vi "TCL Get Valid Baseline.vi"(1 "RFMod (kHz)":i32, 2 "RFFreq (MHz)":dbl format="%.2f", 3 "Baseline Event #":i32) -> (0 "Baseline":dbl[](array[numeric]) format="%.2f")   [LabVIEW 2009]
doc: "This VI looks up the requested event number and then compares its rf frequency and modulation with the input values. If the event is found, and if the frequency and modulation match, the raw signal of the baseline is returned. Otherwise, an empty array is returned."
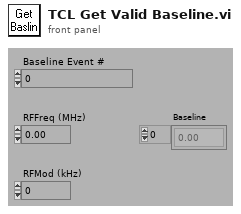
[diagram p1: front panel]
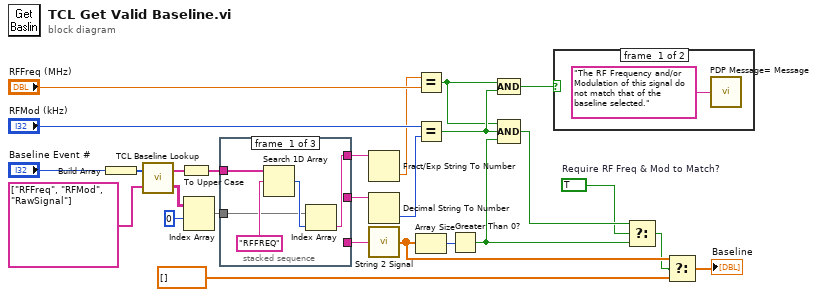
[diagram p0: block diagram]
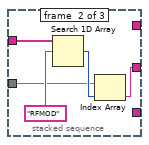
[diagram p3: hidden frame]
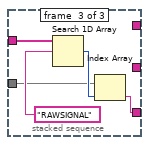
[diagram p4: hidden frame]
diagram:
  w4 = TRUE  # Require RF Freq & Mod to Match?
  n1 = Build Array("Baseline Event #") -> (w13:i32[])
  n2 = call "TCL Baseline Lookup.vi"("Fragments Desired"=string[] ["RFFreq", "RFMod", "RawSignal"], "Events Requested"=w13) -> ("Data"=w12:string[][], "Fragments Returned"=w11:string[])
  n3 = To Upper Case(1:w11) -> (0:w25:string[])
  n4 = Index Array(array=w12, index (row)=0) -> (element=w22:string[])  [unwired: 1 in]
  n5 = stacked-sequence {
    tunnel: w25 -> [w31 w36 w41]
    tunnel: w22 -> [w28 w33 w38]
    tunnel: [w27 _ _] -> w21
    tunnel: [_ w32 _] -> w23
    tunnel: [_ _ w37] -> w24
    frame #0 {
      n6 = Search 1D Array(1D array=w31, element="RFFREQ") -> (index of element=w29:i32)  [unwired: 1 in]
      n7 = Index Array(array=w28, index=w29) -> (element=w27:string)
    }
    frame #1 {
      n8 = Search 1D Array(1D array=w36, element="RFMOD") -> (index of element=w34:i32)  [unwired: 1 in]
      n9 = Index Array(array=w33, index=w34) -> (element=w32:string)
    }
    frame #2 {
      n10 = Search 1D Array(1D array=w41, element="RAWSIGNAL") -> (index of element=w39:i32)  [unwired: 1 in]
      n11 = Index Array(array=w38, index=w39) -> (element=w37:string)
    }
  }
  n12 = Fract/Exp String To Number(string=w21) -> (number=w16:dbl)  [unwired: 3 in, 1 out]
  n13 = Decimal String To Number(string=w23) -> (number=w15:i32)  [unwired: 2 in, 1 out]
  n14 = call "String 2 Signal.vi"("String"=w24) -> ("Signal"=w9:dbl[])
  n15 = Equal?(x=w16, y="RFFreq (MHz)") -> (x = y?=w2:bool)
  n16 = Equal?(x="RFMod (kHz)", y=w15) -> (x = y?=w3:bool)
  n17 = Array Size(array=w9) -> (size(s)=w8:i32)
  n18 = Greater Than 0?(x=w8) -> (x > 0?=w7:bool)
  n19 = Compound Arithmetic op=AND(w2, w3) -> (w1:bool)
  n20 = Compound Arithmetic op=AND(w2, w3, w7) -> (w6:bool)
  n21 = case shown="False" w1 {
    frame #0 {
      n22 = call "PDP Message= Message.vi"("Message"="The RF Frequency and/or Modulation of this signal do not match that of the baseline selected.") -> ()
    }
    frame #1 {
    }
  }
  n23 = Select(t=w6, s=w4, f=w7) -> (s? t:f=w5:bool)
  n24 = Select(t=w9, s=w5, f=dbl[] []) -> (s? t:f=→"Baseline":dbl[])
